vi "Read FPGA VI Reference Out.vi"(8 "error in (no error)":errorcluster, 11 "nCRD in":refnum<class "nCRD.lvclass">) -> (0 "error out":errorcluster, 2 "FPGA VI Reference Out":T1, 3 "nCRD out":refnum<class "nCRD.lvclass">)   [LabVIEW 2013, in "nCRD.lvclass"]
uses:
  nCRD.lvclass
  FPGA Ref.ctl
  nCRD.lvclass/nCRD.ctl
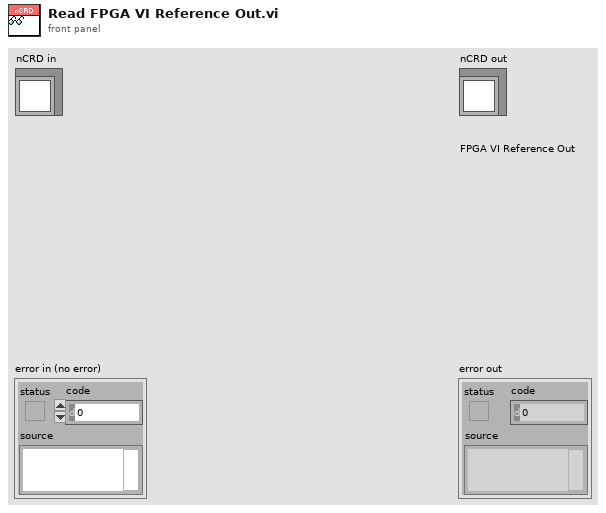
[diagram p1: front panel]
types:
  T1 = typedef "FPGA Ref.ctl" = refnum<k20>
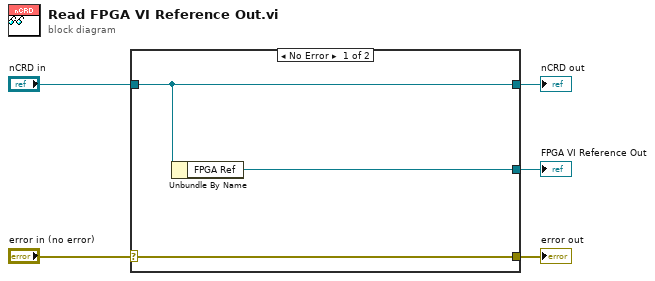
[diagram p0: block diagram]
diagram:
  n1 = case shown="No Error" "error in (no error)" {
    selector: "error in (no error)" -> [w8 w9]
    tunnel: [w8 w9] -> w4
    tunnel: [w7 w10] -> w2
    tunnel: "nCRD in" -> [w7 w10]
    tunnel: [w6 _] -> w1
    frame No Error {
      n2 = Unbundle By Name(w7) -> ("FPGA Ref"=w6:T1)
    }
    frame Error {
    }
  }
  "error out" <- w4
  "nCRD out" <- w2
  "FPGA VI Reference Out" <- w1
